vi "Untitled 1.vi"() -> ()   [LabVIEW 2016]
uses:
  <vilib>/TagLibrary/Create Tag (Double).vi
  <vilib>/TagLibrary/Write (Double).vi
  <vilib>/TagLibrary/Close Tag (Single).vi
  <vilib>/TagLibrary/TagLibrary.lvlib
  <resource>/objmgr/niTag.rc
panel:
  out "error out":errorcluster
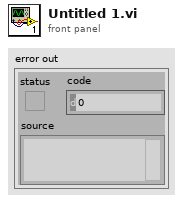
[diagram p1: front panel]
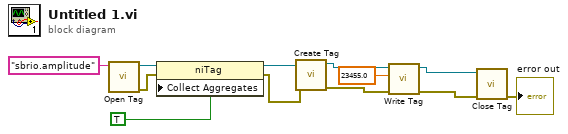
[diagram p0: block diagram]
diagram:
  n1 = call <vilib>:"Open Tag.vi"("tag path"="sbrio.amplitude") -> ("error out"=w11:errorcluster, "tag reference out"=w6:refnum<k21>)  [unwired: 9 in]
  n2 = property class="niTag"(reference=w6, error in=w11, "Collect Aggregates"=TRUE) -> (reference out=w9:refnum<k21>, error out=w12:errorcluster)
  n3 = call-poly <vilib>:"Create Tag.vi"("error in (no error)"=w12, "tag reference in"=w9) -> ("error out"=w5:errorcluster, "tag reference out"=w8:refnum<k21>)  [unwired: 8 in]
  n4 = call-poly <vilib>:"Write Tag.vi"("error in (no error)"=w5, "double"=23455.0, "tag reference in"=w8) -> ("error out"=w4:errorcluster, "tag reference out"=w7:refnum<k21>)  [unwired: 7 in]
  n5 = call-poly <vilib>:"Close Tag.vi"("error in (no error)"=w4, "tag reference"=w7) -> ("error out"=→"error out":errorcluster)  [unwired: 9 in]
